vi "Read Array.vi"   [LabVIEW 2020, in "NH Research Regenerative Test Series.lvlib"]
doc: "Initiates a measurement and returns an array containing the instantaneous input voltage or current for the specified phase.\n\nWaveforms are captured with every initiated measurement based on the Set Aperture Length.vi and Set Number of Samples.vi commands."
uses:
  Drivers-NHR-9200/NHR/NH Research Regenerative Test Series.lvlib
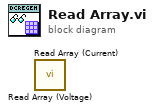
[diagram p0: block diagram]
diagram:
  n1 = call "Read Array (Voltage).vi"() -> ()  [unwired: 13 in, 3 out]
  n2 = call "Read Array (Current).vi"() -> ()  [unwired: 13 in, 3 out]
